vi "Timing.Iteration.Set.vi"(8 "error in (no error)":errorcluster, 10 "iteration":u64=1, 11 "Timing in":refnum<class "Timing.lvclass">) -> (0 "error out":errorcluster, 3 "Timing out":refnum<class "Timing.lvclass">)   [LabVIEW 2017, in "DSF.Engine.lvlib" / "Timing.lvclass"]
uses:
  Timing.lvclass
  Timing.lvclass/Timing.ctl
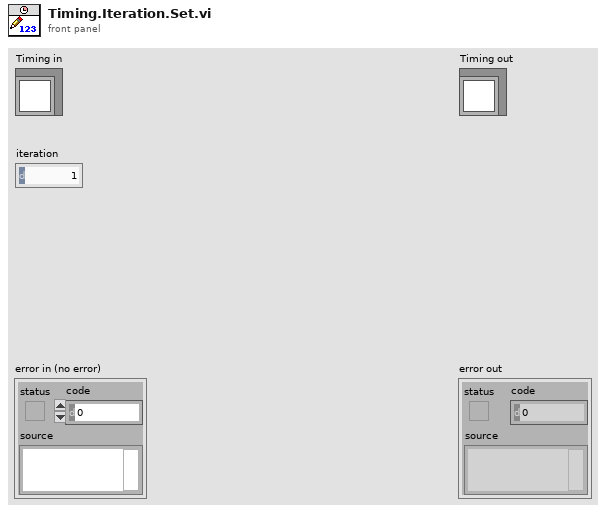
[diagram p1: front panel]
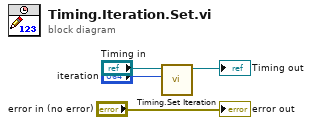
[diagram p0: block diagram]
diagram:
  n1 = call "Timing.Set Iteration.vi"("Iteration"="iteration", "Timing in"="Timing in") -> ("Timing out"=→"Timing out":refnum<class "Timing.lvclass">)  [unwired: 9 in]
  "error out" <- "error in (no error)"
